vi "lab2_1.vi"(1 "x":dbl) -> (0 "sin(x)":dbl)   [LabVIEW 2015]
uses:
  <vilib>/gmath/NI_Gmath.lvlib
panel:
  out "sin(x)2":dbl
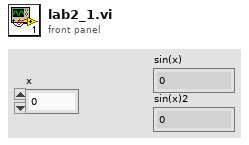
[diagram p1: front panel]
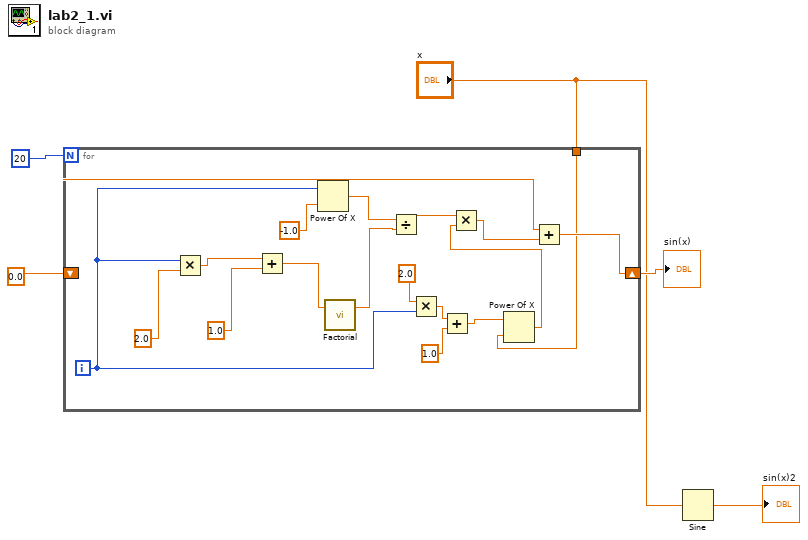
[diagram p0: block diagram]
diagram:
  n1 = for {
    N: 20 -> [_]
    shift-right: [w11] -> w4
    shift-left: 0.0 -> [w13]
    tunnel: "x" -> [w8]
    i -> [w6]
    n2 = Multiply(x=w6, y=2.0) -> (x*y=w22:dbl)
    n3 = Add(x=w22, y=1.0) -> (x+y=w20:dbl)
    n4 = Power Of X(1:-1.0, 2:w6) -> (0:w17:dbl)
    n5 = call <vilib>:"Factorial.vi"("n"=w20) -> ("n!"=w19:dbl)  [unwired: 2 in]
    n6 = Divide(x=w17, y=w19) -> (x/y=w16:dbl)
    n7 = Multiply(x=2.0, y=w6) -> (x*y=w12:dbl)
    n8 = Add(x=w12, y=1.0) -> (x+y=w9:dbl)
    n9 = Power Of X(1:w8, 2:w9) -> (0:w7:dbl)
    n10 = Multiply(x=w16, y=w7) -> (x*y=w10:dbl)
    n11 = Add(x=w13, y=w10) -> (x+y=w11:dbl)
  }
  "sin(x)" <- w4
  n12 = Sine(x="x") -> (sin(x)=→"sin(x)2":dbl)
